vi "Control Drive with Limelight.vi"(9 "X-DriveAuto":dbl, 11 "Y-DriveAuto":dbl) -> ()   [LabVIEW 2020]
uses:
  Framework/Robot Global Data.vi
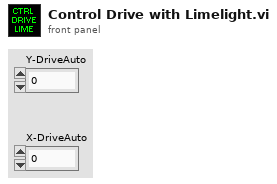
[diagram p1: front panel]
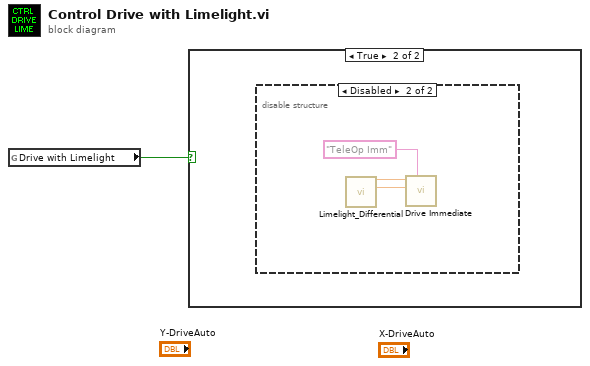
[diagram p0: block diagram]
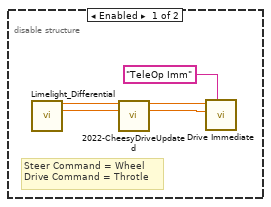
[diagram p3: hidden frame]
diagram:
  n1 = global read "Robot Global Data.vi" "Drive with Limelight"() -> (w1:bool)
  n2 = case shown="True" w1 {
    frame False {
    }
    frame True {
      n3 = disable-structure shown="Disabled" {
        frame Enabled {
          # "Steer Command = Wheel\nDrive Command = Throtle"
          n4 = call "Limelight_Differential.vi"() -> ("SteerCommand"=w2:dbl, "DriveCommand"=w3:dbl)  [unwired: 8 in, 1 out]
          n5 = call "2022-CheesyDriveUpdated.vi"("Throttle"=w3, "Wheel"=w2) -> ("Left PWM"=w5:dbl, "Right PWM"=w4:dbl)  [unwired: 12 in]
          n6 = call "Drive Immediate.vi"("Description"="TeleOp Imm", "Right Setpoint"=w4, "Left Setpoint"=w5) -> ()  [unwired: 8 in, 1 out]
        }
        frame Disabled {
          n7 = call "Limelight_Differential.vi"() -> ("SteerCommand"=w7:dbl, "DriveCommand"=w8:dbl)  [unwired: 8 in, 1 out]
          n8 = call "Drive Immediate.vi"("Description"="TeleOp Imm", "Right Setpoint"=w7, "Left Setpoint"=w8) -> ()  [unwired: 8 in, 1 out]
        }
      }
    }
  }
